vi "Generate Filepath.vi"(9 "File Name":string="PressureData", 11 "Relative Path or Folder":path=path "Data") -> (0 "Date & Time":string, 1 "Log File Name":string, 3 "File Path Output":path)   [LabVIEW 2021]
uses:
  <vilib>/MakerHub/Toolbox/LMH-Toolbox.lvlib
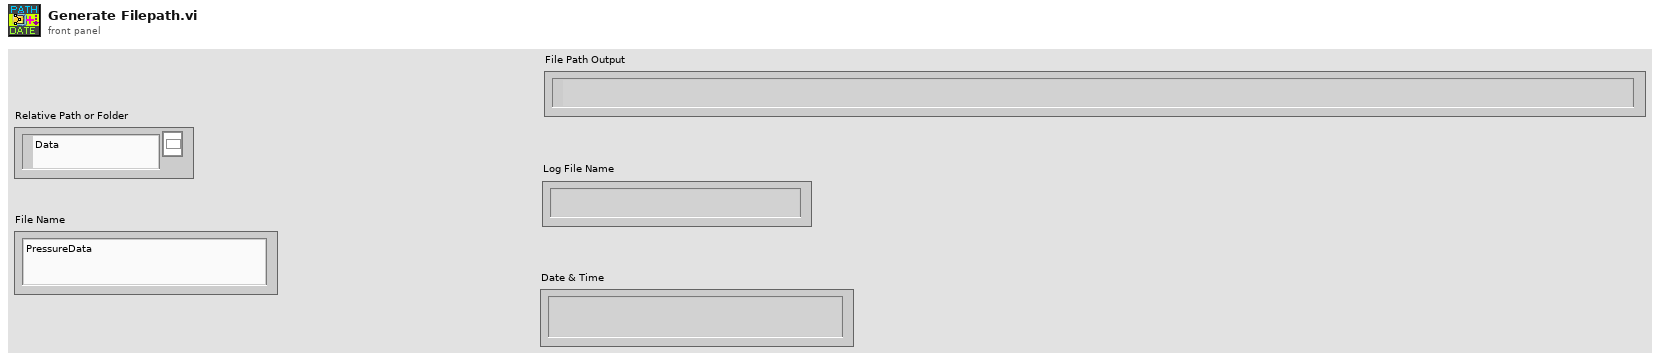
[diagram p1: front panel]
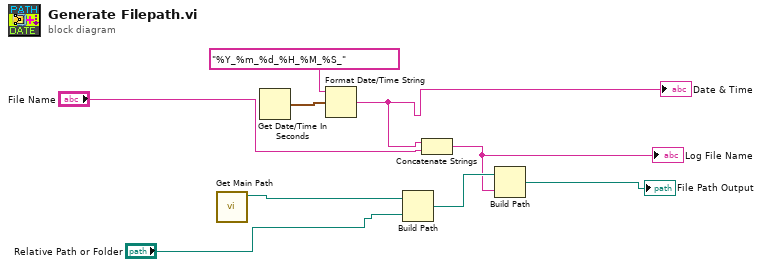
[diagram p0: block diagram]
diagram:
  n1 = call <vilib>:"Get Main Path.vi"() -> ("Main Dir"=w3:path)  [unwired: 9 in, 2 out]
  n2 = Get Date/Time In Seconds() -> (seconds since 1Jan1904=w5:timestamp)
  n3 = Format Date/Time String(time format string (%c)="%Y_%m_%d_%H_%M_%S_", seconds (now)=w5) -> (date/time string=w6:string)  [unwired: 1 in]
  "Date & Time" <- w6
  n4 = Build Path(base path=w3, name or relative path="Relative Path or Folder") -> (appended path=w8:path)
  n5 = Concatenate Strings(w6, "File Name") -> (w7:string)
  "Log File Name" <- w7
  n6 = Build Path(base path=w8, name or relative path=w7) -> (appended path=→"File Path Output":path)
